vi "Circle interpolation.vi"(2 "Yf":i32=16, 3 "Y0":i32=1, 4 "Xf":i32=1, 5 "X0":i32=16) -> (0 "Y array":i32[](array[numeric])=[1, 2, 2, 3, 4, 5, 6, 7, 7, 8, 9, 9, 10, 11, 11, 12, 12, 13, 13, 14, 14, 14, 15, 15, 15, 16, 16, 16, 16, 16, 16], 1 "X array":i32[](array[numeric])=[16, 16, 15, 15, 15, 15, 15, 15, 14, 14, 14, 13, 13, 13, 12, 12, 11, 11, 10, 10, 9, 8, 8, 7, 6, 6, 5, 4, 3, 2, 1])   [LabVIEW 2019]
panel:
  out "XY Graph":cluster{i32[], i32[]}(graph)={[16, 16, 15, 15, 15, 15, 15, 15, 14, 14, 14, 13, 13, 13, 12, 12, 11, 11, 10, 10, 9, 8, 8, 7, 6, 6, 5, 4, 3, 2, 1], [1, 2, 2, 3, 4, 5, 6, 7, 7, 8, 9, 9, 10, 11, 11, 12, 12, 13, 13, 14, 14, 14, 15, 15, 15, 16, 16, 16, 16, 16, 16]}
  # "Начальная точка"
  # "Конечная точка"
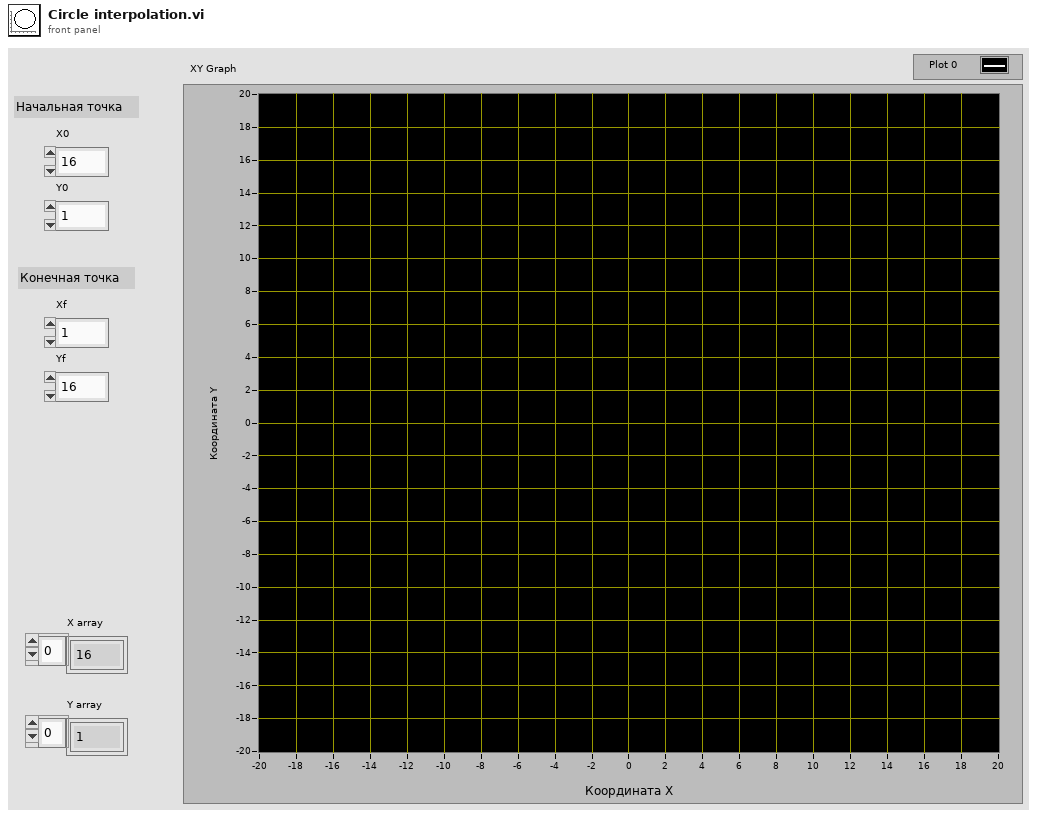
[diagram p1: front panel]
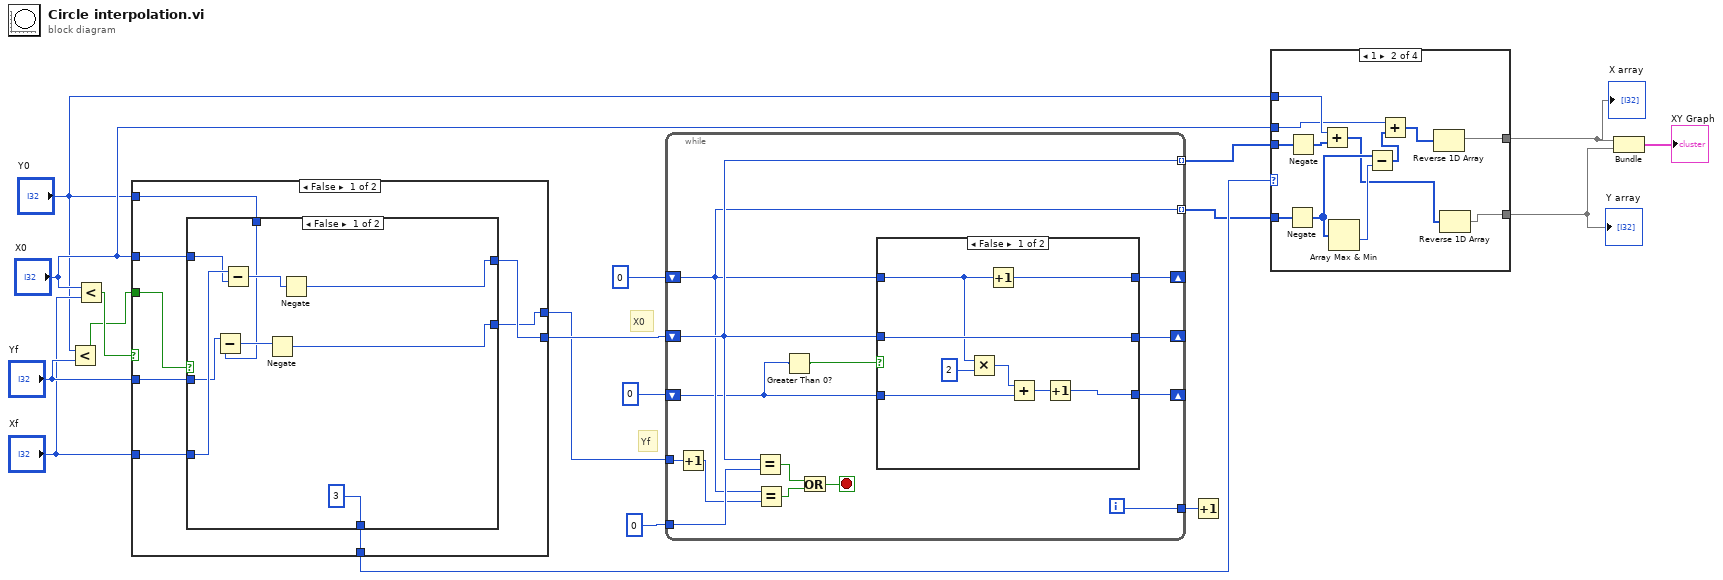
[diagram p0: block diagram]
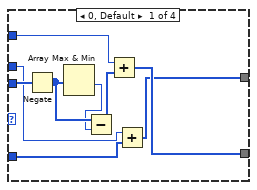
[diagram p2: hidden frame]
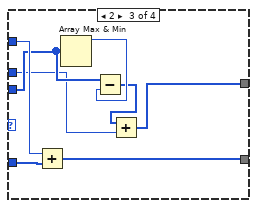
[diagram p3: hidden frame]
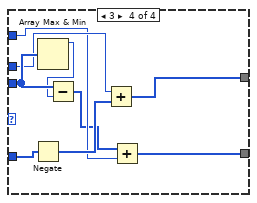
[diagram p4: hidden frame]
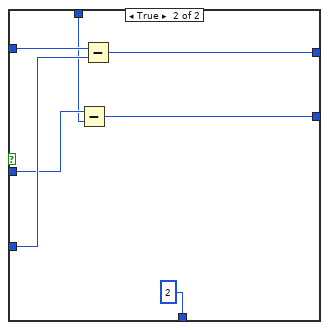
[diagram p5: hidden frame]
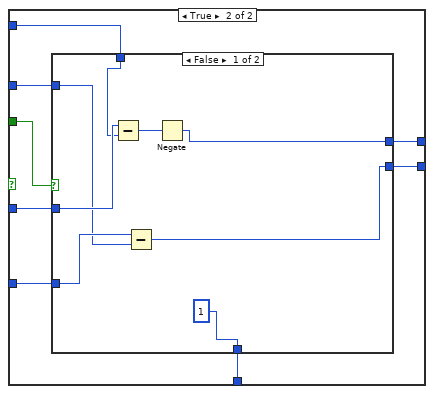
[diagram p6: hidden frame]
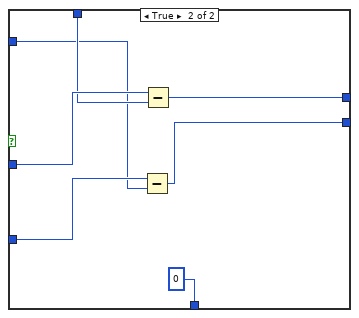
[diagram p7: hidden frame]
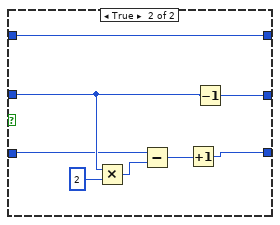
[diagram p8: hidden frame]
diagram:
  # "Yf"
  # "X0"
  n1 = Less?(x="Y0", y="Yf") -> (x < y?=w9:bool)
  n2 = Less?(x="X0", y="Xf") -> (x < y?=w10:bool)
  n3 = case shown="False" w10 {
    tunnel: w9 -> [w26 w50]
    tunnel: [w25 w49] -> w8
    tunnel: "Yf" -> [w22 w48]
    tunnel: "Y0" -> [w21 w47]
    tunnel: "Xf" -> [w23 w46]
    tunnel: "X0" -> [w24 w45]
    tunnel: [w20 w44] -> w12
    tunnel: [w19 w43] -> w11
    frame False {
      n4 = case shown="False" w26 {
        tunnel: [3 2] -> w25
        tunnel: w24 -> [w31 w41]
        tunnel: w23 -> [w32 w40]
        tunnel: w22 -> [w30 w39]
        tunnel: w21 -> [w29 w38]
        tunnel: [w28 w37] -> w20
        tunnel: [w27 w36] -> w19
        frame False {
          n5 = Subtract(x=w30, y=w29) -> (x-y=w34:i32)
          n6 = Subtract(x=w32, y=w31) -> (x-y=w35:i32)
          n7 = Negate(x=w34) -> (-x=w27:i32)
          n8 = Negate(x=w35) -> (-x=w28:i32)
        }
        frame True {
          n9 = Subtract(x=w39, y=w38) -> (x-y=w36:i32)
          n10 = Subtract(x=w41, y=w40) -> (x-y=w37:i32)
        }
      }
    }
    frame True {
      n11 = case shown="False" w50 {
        tunnel: [1 0] -> w49
        tunnel: w48 -> [w56 w64]
        tunnel: w47 -> [w55 w63]
        tunnel: w46 -> [w54 w62]
        tunnel: w45 -> [w53 w61]
        tunnel: [w51 w60] -> w44
        tunnel: [w52 w59] -> w43
        frame False {
          n12 = Subtract(x=w56, y=w55) -> (x-y=w58:i32)
          n13 = Subtract(x=w54, y=w53) -> (x-y=w51:i32)
          n14 = Negate(x=w58) -> (-x=w52:i32)
        }
        frame True {
          n15 = Subtract(x=w62, y=w61) -> (x-y=w60:i32)
          n16 = Subtract(x=w64, y=w63) -> (x-y=w59:i32)
        }
      }
    }
  }
  n17 = while {
    shift-right: [w75] -> _
    shift-left: 0 -> [w71]
    shift-right: [w73] -> _
    shift-left: w12 -> [w72]
    tunnel: w11 -> [w67]
    tunnel: 0 -> [w76]
    shift-right: [w74] -> _
    shift-left: 0 -> [w68]
    tunnel: [w72] -> w6 mode=indexing
    tunnel: [w71] -> w7 mode=indexing
    tunnel: [w70] -> w17
    i -> [w70]
    stop <- w79 stop-if-true
    n18 = Increment(x=w67) -> (x+1=w66:i32)
    n19 = Equal?(x=w72, y=w76) -> (x = y?=w77:bool)
    n20 = Equal?(x=w71, y=w66) -> (x = y?=w78:bool)
    n21 = Greater Than 0?(x=w68) -> (x > 0?=w69:bool)
    n22 = Or(x=w77, y=w78) -> (x .or. y?=w79:bool)
    n23 = case shown="False" w69 {
      tunnel: [w80 w88] -> w74
      tunnel: w68 -> [w83 w89]
      tunnel: w72 -> [w86 w91]
      tunnel: [w87 w92] -> w75
      tunnel: w71 -> [w85 w92]
      tunnel: [w86 w90] -> w73
      frame False {
        n24 = Multiply(x=w85, y=2) -> (x*y=w82:i32)
        n25 = Increment(x=w85) -> (x+1=w87:i32)
        n26 = Add(x=w82, y=w83) -> (x+y=w81:i32)
        n27 = Increment(x=w81) -> (x+1=w80:i32)
      }
      frame True {
        n28 = Multiply(x=w91, y=2) -> (x*y=w95:i32)
        n29 = Subtract(x=w89, y=w95) -> (x-y=w93:i32)
        n30 = Increment(x=w93) -> (x+1=w88:i32)
        n31 = Decrement(x=w91) -> (x-1=w90:i32)
      }
    }
  }
  n32 = Increment(x=w17) -> ()  [unwired: 1 out]
  n33 = case shown="1" w8 {
    tunnel: w7 -> [w97 w115 w124 w131]
    tunnel: w6 -> [w104 w116 w120 w133]
    tunnel: "X0" -> [w98 w109 w117 w129]
    tunnel: "Y0" -> [w101 w111 w123 w126]
    tunnel: [w96 w108 w119 w130] -> w3
    tunnel: [w99 w106 w122 w128] -> w2
    frame 0, Default {
      n34 = Negate(x=w104) -> (-x=w103:i32[])
      n35 = Array Max & Min(array=w103) -> (min value=w102:i32)  [unwired: 3 out]
      n36 = Subtract(x=w103, y=w102) -> (x-y=w100:i32[])
      n37 = Add(x=w101, y=w100) -> (x+y=w99:i32[])
      n38 = Add(x=w98, y=w97) -> (x+y=w96:i32[])
    }
    frame 1 {
      n39 = Negate(x=w115) -> (-x=w114:i32[])
      n40 = Negate(x=w116) -> (-x=w112:i32[])
      n41 = Add(x=w111, y=w112) -> (x+y=w105:i32[])
      n42 = Array Max & Min(array=w114) -> (min value=w113:i32)  [unwired: 3 out]
      n43 = Subtract(x=w114, y=w113) -> (x-y=w110:i32[])
      n44 = Add(x=w109, y=w110) -> (x+y=w107:i32[])
      n45 = Reverse 1D Array(array=w107) -> (reversed array=w108:i32[])
      n46 = Reverse 1D Array(array=w105) -> (reversed array=w106:i32[])
    }
    frame 2 {
      n47 = Add(x=w123, y=w124) -> (x+y=w122:i32[])
      n48 = Array Max & Min(array=w120) -> (max value=w121:i32)  [unwired: 3 out]
      n49 = Subtract(x=w120, y=w121) -> (x-y=w118:i32[])
      n50 = Add(x=w118, y=w117) -> (x+y=w119:i32[])
    }
    frame 3 {
      n51 = Negate(x=w131) -> (-x=w127:i32[])
      n52 = Array Max & Min(array=w133) -> (max value=w132:i32)  [unwired: 3 out]
      n53 = Subtract(x=w133, y=w132) -> (x-y=w125:i32[])
      n54 = Add(x=w129, y=w127) -> (x+y=w130:i32[])
      n55 = Add(x=w125, y=w126) -> (x+y=w128:i32[])
    }
  }
  "X array" <- w3
  "Y array" <- w2
  n56 = Bundle(w3, w2) -> (→"XY Graph":cluster{i32[], i32[]})  [unwired: 1 in]
